vi "UI Initialize.vi"(8 "error in (no error)":errorcluster, 11 "User Interface References":T1={"This VI"=refnum, "User Interace Plugin"=refnum, "UI Picture Container References"={"Header Image"=refnum, "Footer Image"=refnum}, "Sliding Menu XControl"=refnum, "Menu Container"=refnum, "UI Configuration Information"={"Space Between Buttons"=3, "Number of Buttons to Show"=6, "Header Image"=path "Images/Blue Background.bmp", "Footer Image"=path "Images/Blue Background.bmp"}, "Header Text"=refnum}) -> (0 "error out":errorcluster, 3 "User Interface References Out":T1={"This VI"=refnum, "User Interace Plugin"=refnum, "UI Picture Container References"={"Header Image"=refnum, "Footer Image"=refnum}, "Sliding Menu XControl"=refnum, "Menu Container"=refnum, "UI Configuration Information"={"Space Between Buttons"=3, "Number of Buttons to Show"=6, "Header Image"=path "Images/Blue Background.bmp", "Footer Image"=path "Images/Blue Background.bmp"}, "Header Text"=refnum})   [LabVIEW 2011]
uses:
  Main Type Definitions/User Interface Type Definitions.ctl
  Main Type Definitions/UI Picture Containers.ctl
  Sliding Menu/Sliding Menu Library/Sliding Menu xControl/Sliding Menu XControl.xctl
  UI Control Definitions/UI Configuration Information.ctl
  <vilib>/Utility/miscctls.llb/LVPositionTypeDef.ctl
  Root Location Global.vi
  <vilib>/Utility/cursorutil.llb/Set Cursor (Icon Pict).vi
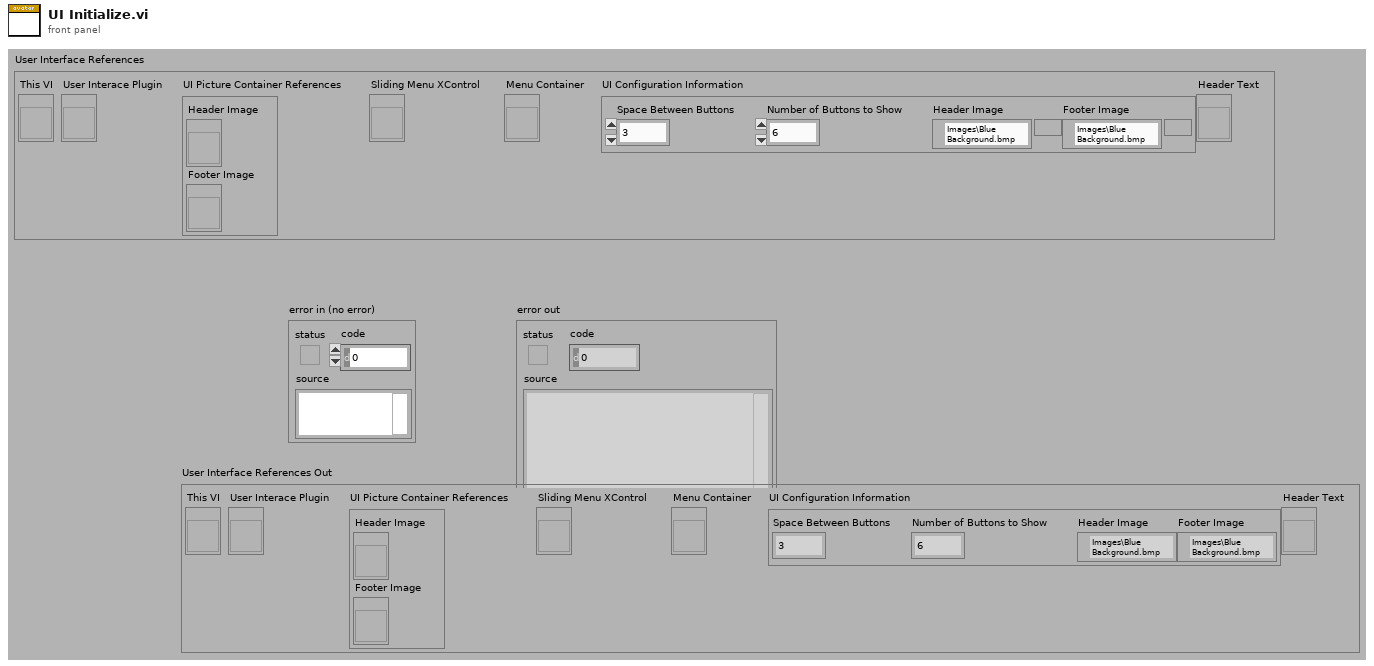
[diagram p1: front panel]
types:
  T1 = typedef "User Interface Type Definitions.ctl" = cluster{"This VI":refnum<vi>, "User Interace Plugin":refnum<vi>, "UI Picture Container References":T2, "Sliding Menu XControl":refnum<vi>, "Menu Container":refnum<vi>, "UI Configuration Information":T3, "Header Text":refnum<vi>}
  T2 = typedef "UI Picture Containers.ctl" = cluster{"Header Image":refnum<vi>, "Footer Image":refnum<vi>}
  T3 = typedef "UI Configuration Information.ctl" = cluster{"Space Between Buttons":i32, "Number of Buttons to Show":i32, "Header Image":path, "Footer Image":path}
  T4 = typedef "LVPositionTypeDef.ctl" = cluster{"Left":i32, "Top":i32}
  T5 = typedef "imagedata.ctl" = cluster{"image type":i32, "image depth":i32, "image":u8[], "mask":u8[], "colors":u32[], "Rectangle":cluster{"left":i16, "top":i16, "right":i16, "bottom":i16}}
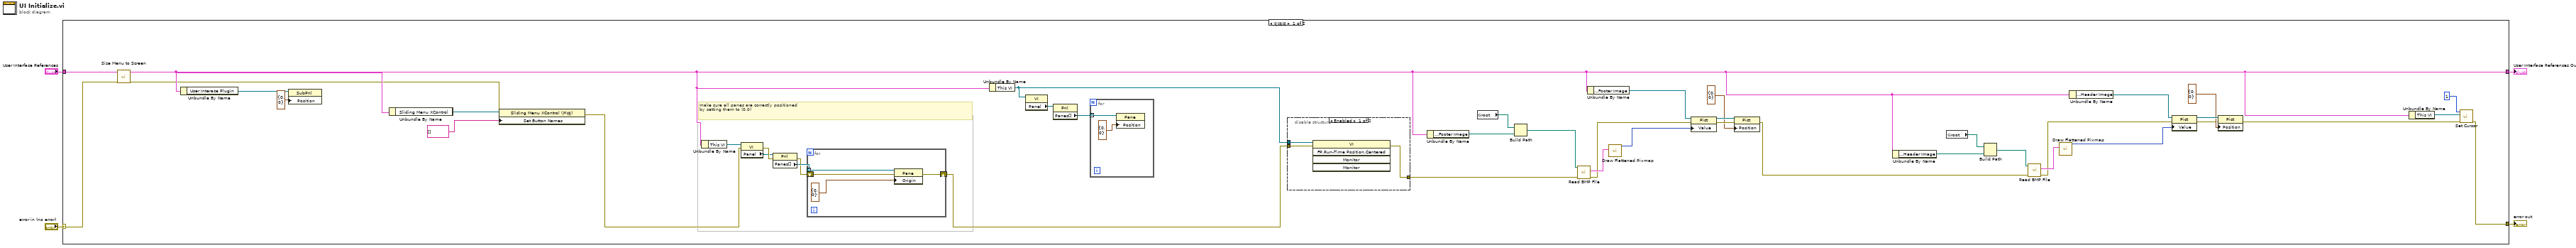
[diagram p0: block diagram]
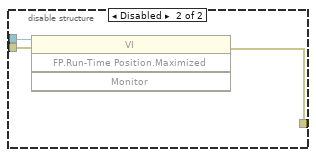
[diagram p2: hidden frame]
diagram:
  n1 = case shown="无错误" "error in (no error)" {
    selector: "error in (no error)" -> [w5 w62]
    tunnel: [w14 w62] -> w4
    tunnel: [w7 w61] -> w1
    tunnel: "User Interface References" -> [w8 w61]
    frame No Error {
      # "make sure all panes are correctly positioned\nby setting them to (0,0)"
      n2 = call "Size Menu to Screen.vi"("error IO"=w5, "User Interface References"=w8) -> ("error out"=w6:errorcluster, "User Interface References Out"=w7:T1)  [unwired: 8 in]
      n3 = Unbundle By Name(w7) -> ("User Interace Plugin"=w13:refnum<vi>)
      n4 = property class="SubPnl"(reference=w13, "Position"=T4 {"Left"=0, "Top"=0}) -> ()  [unwired: 1 in, 2 out]
      n5 = Unbundle By Name(w7) -> ("Sliding Menu XControl"=w42:refnum<vi>)
      n6 = property class="Sliding Menu XControl (严格)"(reference=w42, error in=w6, "Set Button Names"=string[] []) -> (error out=w28:errorcluster)  [unwired: 1 out]
      n7 = Unbundle By Name(w7) -> ("This VI"=w48:refnum<vi>)
      n8 = property class="VI"(reference=w48, error in=w28) -> (error out=w47:errorcluster, "Panel"=w46:refnum<vi>)  [unwired: 1 out]
      n9 = property class="Pnl"(reference=w46, error in=w47) -> (error out=w44:errorcluster, "Panes[]"=w45:refnum<vi>[])  [unwired: 1 out]
      n10 = for {
        tunnel: w45 -> [w60] mode=indexing
        shift-right: [w57] -> w43
        shift-left: w44 -> [w58]
        n11 = property class="Pane"(reference=w60, error in=w58, "Origin"=T4 {"Left"=0, "Top"=0} ("Position")) -> (error out=w57:errorcluster)  [unwired: 1 out]
      }
      n12 = Unbundle By Name(w7) -> ("This VI"=w11:refnum<vi>)
      n13 = property class="VI"(reference=w11) -> ("Panel"=w10:refnum<vi>)  [unwired: 1 in, 2 out]
      n14 = property class="Pnl"(reference=w10) -> ("Panes[]"=w9:refnum<vi>[])  [unwired: 1 in, 2 out]
      n15 = for {
        tunnel: w9 -> [w50] mode=indexing
        n16 = property class="Pane"(reference=w50, "Position"=T4 {"Left"=0, "Top"=0}) -> ()  [unwired: 1 in, 2 out]
      }
      n17 = disable-structure shown="Enabled" {
        disable-tunnel: [w53 w54] -> w22
        disable-tunnel: w11 -> [w52 w56]
        disable-tunnel: w43 -> [w51 w55]
        frame Enabled {
          n18 = invoke class="VI" method="FP.Run-Time Position.Centered"(reference=w52, error in=w51) -> (error out=w53:errorcluster)  [unwired: 3 in, 4 out]
        }
        frame Disabled {
          n19 = invoke class="VI" method="FP.Run-Time Position.Maximized"(reference=w56, error in=w55) -> (error out=w54:errorcluster)  [unwired: 2 in, 3 out]
        }
      }
      n20 = Unbundle By Name(w7) -> ("UI Configuration Information.Footer Image"=w19:path)
      n21 = global read "Root Location Global.vi" "root"() -> (w20:path)
      n22 = Build Path(base path=w20, name or relative path=w19) -> (appended path=w18:path)
      n23 = call <vilib>:"Read BMP File.vi"("error in (no error)"=w22, "path to BMP file"=w18) -> ("error out"=w27:errorcluster, "image data"=w41:T5)  [unwired: 7 in, 1 out]
      n24 = Unbundle By Name(w7) -> ("UI Picture Container References.Footer Image"=w32:refnum<vi>)
      n25 = call <vilib>:"Draw Flattened Pixmap.vi"("image data"=w41) -> ("new picture"=w33:picture)  [unwired: 8 in]
      n26 = property class="Pict"(reference=w32, error in=w27, "Value"=w33) -> (reference out=w35:refnum<vi>, error out=w36:errorcluster)
      n27 = property class="Pict"(reference=w35, error in=w36, "Position"=T4 {"Left"=0, "Top"=0}) -> (error out=w21:errorcluster)  [unwired: 1 out]
      n28 = Unbundle By Name(w7) -> ("UI Configuration Information.Header Image"=w15:path)
      n29 = global read "Root Location Global.vi" "root"() -> (w17:path)
      n30 = Build Path(base path=w17, name or relative path=w15) -> (appended path=w16:path)
      n31 = call <vilib>:"Read BMP File.vi"("error in (no error)"=w21, "path to BMP file"=w16) -> ("error out"=w24:errorcluster, "image data"=w25:T5)  [unwired: 7 in, 1 out]
      n32 = call <vilib>:"Draw Flattened Pixmap.vi"("image data"=w25) -> ("new picture"=w23:picture)  [unwired: 8 in]
      n33 = Unbundle By Name(w7) -> ("UI Picture Container References.Header Image"=w26:refnum<vi>)
      n34 = property class="Pict"(reference=w26, error in=w24, "Value"=w23) -> (reference out=w40:refnum<vi>, error out=w38:errorcluster)
      n35 = property class="Pict"(reference=w40, error in=w38, "Position"=T4 {"Left"=0, "Top"=0}) -> (error out=w37:errorcluster)  [unwired: 1 out]
      n36 = Unbundle By Name(w7) -> ("This VI"=w30:refnum<vi>)
      n37 = call-poly <vilib>:"Set Cursor.vi"("error in (no error)"=w37, "VI reference (current VI)"=w30, "icon"=u16 1) -> ("error out"=w14:errorcluster)  [unwired: 7 in, 1 out]
    }
    frame Error {
    }
  }
  "error out" <- w4
  "User Interface References Out" <- w1
